vi "Setup.vi"(10 "Setup":T1, 11 "TEMPLATE Actor in":refnum<class "TEMPLATE Actor.lvclass">) -> (0 "Error out":errorcluster, 3 "TEMPLATE Actor out":refnum<class "TEMPLATE Actor.lvclass">)   [LabVIEW 2025, in "_Template.lvlib" / "Templates.lvlib" / "TEMPLATE Actor.lvlib" / "TEMPLATE Actor.lvclass"]
uses:
  TEMPLATE Actor.lvclass
  TEMPLATE Actor.lvclass/TEMPLATE Actor.ctl
  jettl/jettl/Actor/Actor/Actor.lvclass
  jettl/jettl/Attributes/Attributes/Attributes.lvclass
  jettl/jettl/Msg/Msg.lvclass
  jettl/jettl/Actor/Msg Set.ctl
  jettl/jettl/Actor/Actor.lvlib
  jettl/jettl/Actor/Setup.ctl
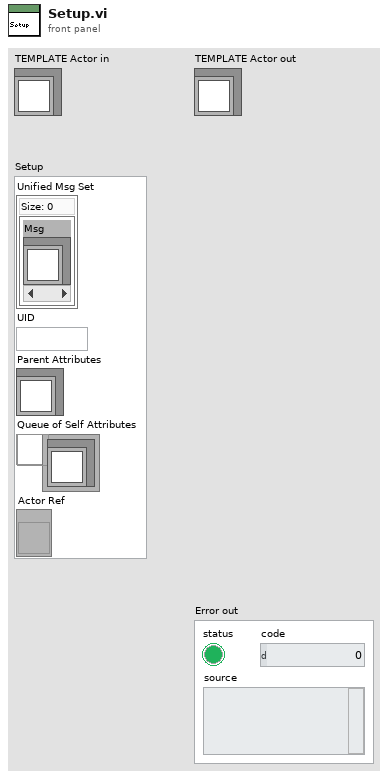
[diagram p1: front panel]
types:
  T1 = typedef "jettl.lvlib/Actor.lvlib/Setup.ctl" = cluster{"Unified Msg Set":T2, "UID":string, "Parent Attributes":refnum<class "Attributes.lvclass">, "Queue of Self Attributes":refnum<queue>, "Actor Ref":refnum<vi>}
  T2 = typedef "jettl.lvlib/Actor.lvlib/Msg Set.ctl" = set{refnum<class "Msg.lvclass">}
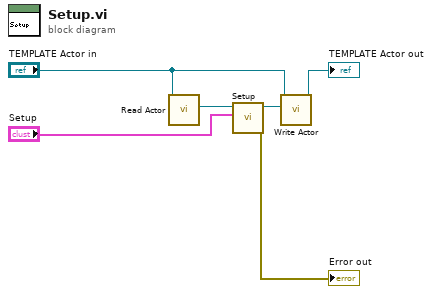
[diagram p0: block diagram]
diagram:
  n1 = call-dynamic "Read Actor.vi"("TEMPLATE Actor in"="TEMPLATE Actor in") -> ("Actor"=w1:refnum<class "Actor.lvclass">)  [unwired: 10 in]
  n2 = call-dynamic "Setup.vi"("Setup"="Setup", "Actor in"=w1) -> ("Error out"=→"Error out":errorcluster, "Actor out"=w2:refnum<class "Actor.lvclass">)  [unwired: 8 in]
  n3 = call-dynamic "Write Actor.vi"("Actor"=w2, "TEMPLATE Actor in"="TEMPLATE Actor in") -> ("TEMPLATE Actor out"=→"TEMPLATE Actor out":refnum<class "TEMPLATE Actor.lvclass">)  [unwired: 9 in]
